vi "MovingDateTrans V1.0 for TCP.vi"(2 "INPUT":dbl[](array[numeric]), 3 "String":string) -> (0 "MOVEING COMMAND":string)   [LabVIEW 2016]
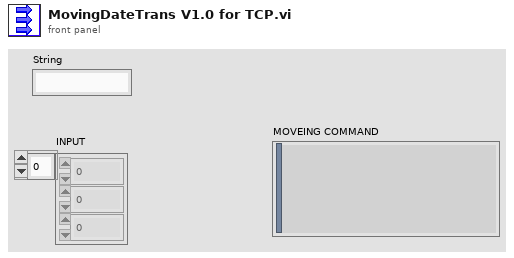
[diagram p1: front panel]
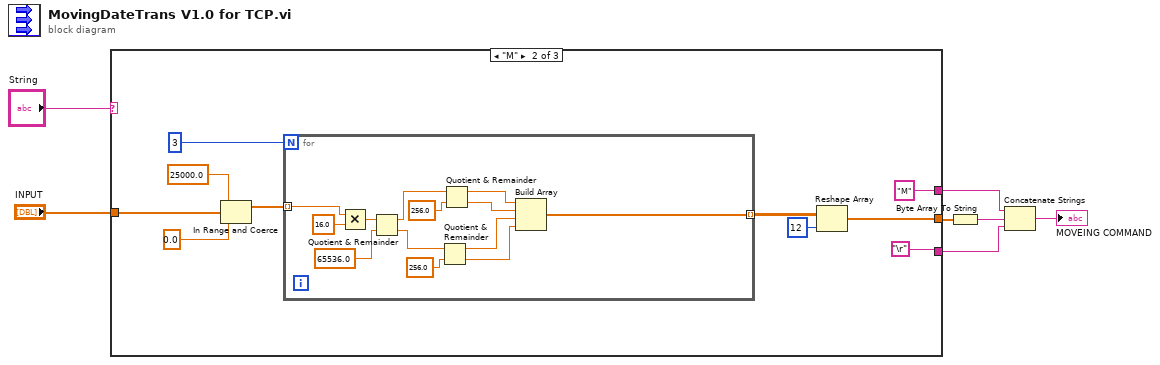
[diagram p0: block diagram]
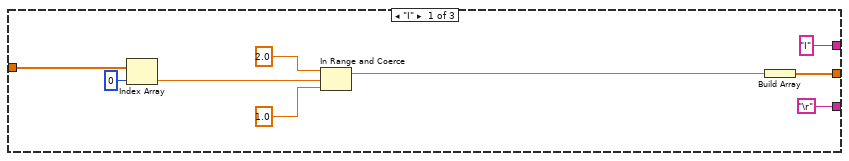
[diagram p2: hidden frame]
diagram:
  n1 = case shown="\"M\"" "String" {
    tunnel: "INPUT" -> [w16 w22 _]
    tunnel: [w11 w18 _] -> w3
    tunnel: ["I" ("string") "M" ("string") _] -> w5
    tunnel: ["\r" "\r" _] -> w1
    frame "I" {
      n2 = Index Array(array=w16, index=0) -> (element=w14:dbl)
      n3 = In Range and Coerce(upper limit=2.0, x=w14, lower limit=1.0) -> (coerced(x)=w10:dbl)  [unwired: 1 out]
      n4 = Build Array(w10) -> (w11:dbl[])
    }
    frame "M" {
      n5 = In Range and Coerce ("判定范围并强制转换")(upper limit=25000.0 ("上限"), x=w22, lower limit=0.0 ("下限")) -> (coerced(x)=w24:dbl[])  [unwired: 1 out]
      n6 = for {
        N: 3 -> [_]
        tunnel: w24 -> [w34] mode=indexing
        tunnel: [w27] -> w21 mode=indexing
        n7 = Multiply(x=w34, y=16.0) -> (x*y=w36:dbl)
        n8 = Quotient & Remainder(x=w36, y=65536.0) -> (x-y*floor(x/y)=w38:dbl, floor(x/y)=w32:dbl)
        n9 = Quotient & Remainder(x=w32, y=256.0) -> (x-y*floor(x/y)=w29:dbl, floor(x/y)=w28:dbl)
        n10 = Quotient & Remainder(x=w38, y=256.0) -> (x-y*floor(x/y)=w31:dbl, floor(x/y)=w30:dbl)
        n11 = Build Array(w31, w30, w29, w28) -> (w27:dbl[])
      }
      n12 = Reshape Array(w21, 12 ("dimension size")) -> (w18:dbl[])
    }
    frame Default {
    }
  }
  n13 = Byte Array To String(unsigned byte array=w3) -> (string=w2:string)
  n14 = Concatenate Strings(w5, w2, w1) -> (→"MOVEING COMMAND":string)
